vi "Identify Autonomous Selection.vi"(9 "Switch Position":string, 11 "Robot Position":T1) -> (3 "Autonomous Selection":string)   [LabVIEW 2017]
uses:
  <vilib>/Rock Robotics/WPI/DriverStation/WPI_DriverStationPositionInfo.ctl
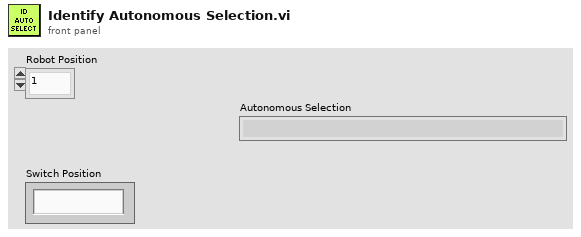
[diagram p1: front panel]
types:
  T1 = typedef "WPI_DriverStationPositionInfo.ctl" = enum16{"1", "2", "3"}
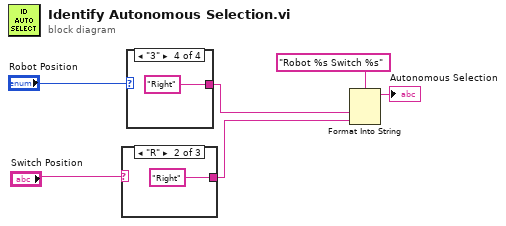
[diagram p0: block diagram]
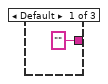
[diagram p2: hidden frame]
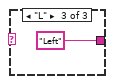
[diagram p3: hidden frame]
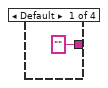
[diagram p4: hidden frame]
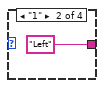
[diagram p5: hidden frame]
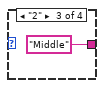
[diagram p6: hidden frame]
diagram:
  n1 = case shown="\"R\"" "Switch Position" {
    tunnel: ["" "Right" "Left"] -> w2
    frame Default {
    }
    frame "R" {
    }
    frame "L" {
    }
  }
  n2 = case shown="\"3\"" "Robot Position" {
    tunnel: ["" "Left" "Middle" "Right"] -> w3
    frame Default {
    }
    frame "1" {
    }
    frame "2" {
    }
    frame "3" {
    }
  }
  n3 = Format Into String(format string="Robot %s Switch %s", w3, w2) -> (resulting string=→"Autonomous Selection":string)  [unwired: 2 in, 1 out]
